vi "UHR-Fleezers Control (host) - Lorentz v5.vi"() -> ()   [LabVIEW 2014] (continued)
0.0016948540928536408, 0.004005193075967077, 0.000630961805097272, 0.0020857235483909497, 0.002248391411474813, 0.0025483315899778513, -0.00014289269800604444, 0.0013990991209830745, 0.002173222163707994, 0.0034697000160164738, 0.002010257683945241, 0.003481043985686529], [0.0018852656320276734, 0.0015715368380061585, 0.0019437671829601755, 0.002470975354509278, 0.0024487910797092428, 0.0007322022696453588, 0.0015475009764890752, 0.0017921866327059758, 0.003058459886432621, 0.0017764067983640703, 0.0025000139148490196, 0.0009623442611020518, 0.0018569165732802914, 0.003310838721775616, 0.00025071352576413444, 0.0036691347962582426, 0.002403046381925506, 0.004055721651469297, 0.002285952907609213, 0.0030062679778400502], [0.0024994380659973843, 0.0026197462346229062, 0.0017527989664171077, 0.0014375842896685127, 0.0033490362530976267, 0.0027052287063586847, 6.381847016474479e-05, 0.0011272327680753905, 0.003454975387457779, 0.004620127122907865, 0.0021178429445671146, 0.004539862151248757, 0.002029684806888378, 0.0013671243967539456, 0.003118446743148983, 0.0010709513970555225, 0.0019090166550763074, 0.002155844648949404, 0.004106378336132433, 0.0010766929367924097], [0.002854938319315421, 0.0038921928444872822, 0.0019246852509770592, 0.001956082424171971, 0.00249396489250124, 0.0024337273809226364, 0.0010765238019800384, 0.002941500719693421, 0.0030759660483101006, 0.0016202953746738819, 0.0017239866140603627, 0.002438327547432977, 0.002786814289877852, 0.002350374795189492, 0.0014284651785432274, 0.0024175263736445143, 0.0017989840672716986, 0.00010277744000073804, 0.0015758938162554312, 0.0015914808231177855], [0.0023379764512881855, 0.0019152406361689915, 0.0023721211744209382, 0.0028072318841611175, 0.00045998972816663626, 0.0019525984204332083, 0.001965702699358644, 0.0032523064679092764, 0.000928270862367026, 0.0025551238347956457, 0.0027235426100884804, 0.0006003323047511277, 0.0024452031525158107, 0.003200615692319165, 0.0031679408338207383, 0.001713752296656085, 0.0029069566496737467, 0.0017760622106257355, 0.0032846637736200987, 0.0014145046584398283], [0.0017413311095229888, 0.002850684453478228, 0.004119312336274303, 0.001376098161794153, 0.0028391954791758406, 0.0023504256794032296, 0.001939098372782241, 0.0009962144963960734, 0.0017508511614465492, 0.0010266285265010658, 0.00317450379791817, 0.002092576486750102, 0.003523745928434037, 0.003362704188893568, 0.0022223282833307503, 0.003285433624934814, 0.0021443498633667525, 0.0006378287745106628, 0.0009042965230192737, 0.004364189912157604], [0.0025684771943308964, 0.003595940600289024, 0.0015386127114892655, 0.002970017638684016, 0.000731008903710616, 0.0015627389249673368, 0.00268734680621615, 0.00033321301039761556, 0.002657761688265375, 0.0018452193301245214, 0.0019648865080461276, 0.00321862929090469, 0.002422721362346656, 0.0036160768033011536, 0.0023323715302130984, 0.0016526314538286777, 0.0033099223028642, 0.0014149263891099, 0.00254445644786201, 0.002714841511848489], [0.00302323496353701, 0.0016076200915618212, 0.001298400361326538, 0.0018074432822074325, 0.0026357010223677386, 0.002293142925429444, 0.001403310979000166, 0.002185113177831846, 0.002789454480226071, 0.0017208525559712065, 0.0017792513529249357, 0.0019822099798379907, 0.0028293142834817267, 0.002262865370925418, 0.001290800627866991, 0.0023298166748236485, 0.0013506602320411689, 0.002143358706259156, 0.0035532369528369174, 0.0017335871199569027], [0.0025192336907101567, 0.0023420394966944366, 0.0018803373952631193, 0.0019133833353522055, 0.0012596720449505453, 0.002147060132875675, 0.0006990538240453468, 0.0021223766921043765, 0.0033568805410328644, 0.0019950947049262504, 0.0021300391805659505, 0.001813624441258409, 0.0011352622065457982, 0.002742817450067307, 0.002825619560905981, 0.0028865080849197105, 0.003418778555540925, 0.0015302210369144652, 0.004455456383213908, 0.0013599469983302684], [-0.0004438837985084353, 0.0028183355707480946, 0.0028130708775573115, 0.0030206214884492544, 3.0807351233010224e-06, 0.00100356141409364, 0.003239142551743778, 0.0028015305417013713, 0.0016360555337629936, 0.0021630034342628546, 0.002737139846047398, 0.0036584890379432007, 0.002471730052534626, 0.0023361339599424456, 0.0029788411839639624, 0.0014442602794432905, 0.0023810759191331154, 0.0012413151489925564, 0.0019023668482100798, 0.002640107429201507], [0.001554782428247715, 0.002954419634687952, 0.0028951557424149637, 0.003310458814954959, 0.002365836700244099, 0.0030819547506098647, 0.0022846439376502706, 0.00043219002702368965, 0.003015949202071104, 0.002476214118282937, 0.0012666534517914985, 0.003753630460609294, 0.0019762301625312097, 0.0024128905675427107, 0.0024715495496260395, 0.0012053557199650255, 0.0030770984437811398, 0.001260030580666012, 0.002103542906975703, 0.003243844033696315], [0.002047169886274074, 0.003135570533130444, 0.003659218345652883, 0.003351918820368115, 0.002638669639842362, 0.0032054173808839705, 0.002728466251491257, 0.002422436287272547, 0.0027550251027393968, 0.0011484124718350213, 0.0024811181138690744, 0.000633754661919369, 0.004103389272200948, 0.002413442590560708, 0.0010161905814301843, 0.0006117013741451642, 0.00043229932014902874, 0.0026398449564406256, 0.002421923707756009, 0.0037337823125722382], [0.003223733537026557, 0.0018388836414569803, 0.0009593646694003638, 0.002150504738108695, 0.002240376826733987, 0.002819775892773071, 0.0023671589694118722, 0.000575767662750824, 0.002985254604568729, 0.0016894905303978737, 0.0022470149983889803, 0.0003279829367159081, 0.0036647064650229947, 0.0034208513812910607, 0.001372326074939035, 0.0012329776908317572, 0.0021677603380249777, 0.002634189260273172, 0.0028446181528041406, 0.00213113583206634], [0.0019954076065657263, 0.0037723924706211747, 0.001706529185397683, 0.002364821147683791, 0.002979725244773599, 0.0025437175845808863, 0.0021453554509108016, 0.004057319159369964, 0.003080980549531066, 0.002721994671347667, 0.0023390951175459806, 0.00256423096986864, 0.0028016019632848403, 0.004136674747509183, 0.0013482163844892154, 0.0025822615725757214, 0.0036704638004895884, 0.0027356369424274387, 0.0026386812531819896, 0.004017865052466032], [0.0024523481698112215, 0.001577397825690218, 0.003482073577677887, 0.0013120929321507693, 0.0023779996424196947, 0.0031885279055957677, 0.0030968142000769574, 0.0008079901646664205, 0.002057639245236158, 0.0014454916165466576, 0.0024913028609758626, 0.0037321652111583048, 0.0017568129726518262, 0.002433957686700396, 0.0013519635336044248, 0.0025583649394570035, 0.0028389004443714833, 0.0022371439658448768, 0.0027243471248494314, 0.0029988024916099377], [0.004482728416008117, 0.002106313095020212, 0.0016966090569018176, 0.002396355324914029, 0.0028921242144040655, 0.0015488778727110483, 0.003087584542752191, 0.0015783381053925663, 0.002107198839582597, 0.002028492535057995, 0.002133558230340132, 0.0033792319972435966, 0.0027693102835735124, 0.0018097134809963325, 0.0018729748671947632, 0.002639158100819596, 0.0020228765137224065, 0.0027609921089093853, 0.0018507896888375831, 0.0037945518126489184], [0.0021563482581923206, 0.0032287318120543937, 0.002708679733426596, 0.001050676702211846, 0.0025215820393785435, 0.0028877563801691696, 0.0019552140449292524, 0.0008869258799717261, 0.00135938852287414, 0.0018791457864769595, 0.0023044366557142164, 0.001505864205337834, 0.002869003954012599, 0.002875615556306393, 0.0002350922247605644, 0.001003648267132261, 0.002356427438894899, 0.0023482204070056395, 0.0030151148802336925, 0.0028427289795750045], [0.0038551731030675492, 0.0032190719566552277, 0.0024841888185482774, 0.0021509928606914825, 0.0019762178118407662, 0.0010938081355370294, 0.0013139616940169843, 0.0021720191912326476, 0.0022752909556785724, 0.001220901184309662, 0.0016582026045028472, 0.0024335127088734292, 0.0024787123106594982, 0.0020212943620039874, 0.0016344163085200308, 0.000406346466621824, 0.0029532673665144445, 0.0024979601850372486, 0.0026392577111319635, 0.004397563792842481], [0.0019392152337034533, 0.0025752001941428933, 0.002375394930020305, 0.0028141695664536765, 0.0030603007029344938, 0.0011131838617945628, 0.002016520759374347, 0.0007694648026350759, 0.0015220876353260865, 0.0007363225146947519, 0.000638103757805431, 0.0021367847621378373, 0.0006798563886399791, 0.0030144489262747447, 0.0012521090204634475, 0.0008366649244029356, 0.0025666821561406115, 0.001756081969563725, 0.0032417664621542308, 0.0027129101328840412], [0.004234965435631261, 0.0028807923900716586, 0.003994864856813696, 0.002228016783386847, 0.0020643224474904383, 0.0032080385730002244, 0.0024267095326168985, 0.0017045994219985895, 0.0004388872799201384, 0.0033081602061115307, 0.001876598014475262, 0.002967363816837642, 0.0014745477365160986, 0.0020882770356405143, 0.0013540441866247209, -0.0006440024187520807, 0.0028524616240076846, 0.0014866404270267755, 0.00212329751615424, 0.0033980422597344436], [0.002443103566818908, 0.0028643225076063544, 0.0026559502913978718, 0.0037632868164488202, 0.002284871036146773, 0.0015618259048538988, 0.0017562004198199274, 0.0013422612594893234, 0.0021296203269845397, 0.0025582835925385674, 0.0014546337054565813, 0.0012911088291717825, 0.0016512241182034806, 0.0022875704433646493, 0.003230826380294793, 0.0017297408349598563, 0.0026936683465980803, 0.0034380066316832677, 0.0020340691324621275, 0.0024417322062178165], [-9.989324566289746e-05, 0.002926244866839386, 0.0012902951621840647, 0.0026901742294294408, 0.0007707616757238599, 0.002362816916091356, 0.001011706400022051, 0.0017386970379252784, 0.0020217996444839735, 0.002564324057587132, 7.627346006863279e-05, 0.0002802241821891143, 0.0026582840805945995, 0.004267218692043419, 0.0008375444339060319, 0.001425992926040155, 0.0018555300552344036, 0.0019526652519745082, 0.0035856622760482276, 0.003574377792936731], [0.0022162866870525226, -9.80488992076956e-05, 0.0025575817989724257, 0.0017415298145425548, 0.0027732403933223874, 0.001805105566650088, 0.003135078437970281, 0.00030140619095551545, 0.002650648973281749, 0.0017502683903315023, 0.0010009292556551102, -0.0001580201494951381, 0.002096695649478786, 0.0023734494130614623, 0.001871656497385907, 0.0010147521269191551, 0.0028769559123858206, 0.001535512363638828, 0.0016771158914974686, 0.0036812015349025297], [0.0032911157382341976, 0.0015937673246648396, 0.0022786049298841506, 0.0016435202933210561, -0.000444139543920988, 0.0010322872285660274, 0.0015058197657779827, 0.0015226621305386731, 0.0013670575927993015, 0.001993129770992985, 0.0024129146141866654, -0.000271958439995209, 0.0032173265132192236, 0.001258442789528919, 0.0017013782876058627, 0.002937335820531526, 0.0020141218387929012, 0.00339081594854371, 0.0023237992039019865, 0.0019362936150417998], [0.0010726759952865783, 0.00383807561043779, 0.0038445499562823364, 0.0037327075782894294, 0.0030324176425392917, 0.000939469808843528, 0.0033586682713470056, 0.0007949762712558317, 0.0026842935481138233, 0.0027066995591428656, 0.001000126612503554, 0.0010644965226183879, 0.0012534863266311373, 0.000971090044070356, 0.0020274176610303746, 0.001313872990779878, 0.004415055089640197, 0.0022069739121942404, 0.000147794314328749, 0.003687654343198644], [0.0013238774283048135, 0.0016832656412011497, 0.002987102709259717, 0.0030815330868127306, 0.0029175865629059517, 0.001487872746945953, 0.0026091093679822507, 0.00135137082614052, 0.0011924192830799123, 0.002261800469194393, 0.000771417004330296, 0.0023250295522089758, 0.0016879132492112036, 0.0019726696926899378, 0.001788107104334166, 0.003862482787623552, 0.0024858537507722227, 0.00385855737054356, 0.0015301935270155484, 0.0031097752029073805], [0.0022271538965262065, 0.002149103591341216, 0.0008579581902112741, 0.0030474920826782247, 0.0032464784941930586, 0.002202404463612722, 0.0028610862175354876, 0.00119149906196459, 0.001159386660592406, 0.0010568905868378246, 0.0016045775757651311, 0.002078856957174876, 0.0031696706950223794, 0.0015400561930039819, 0.0018392034125027834, 0.0019016707318218183, 0.0025078250875444456, 0.0021647130900559666, 0.0006667868013903893, 0.002689612407972146], [0.003174915343868663, 0.0017082274160115402, 0.0004799123732484494, 0.002356906409014597, 0.002454123557174727, 0.0019283029529754366, 0.0005167238834184597, 0.0010390784903798918, 0.0022056908793985446, 0.0027450940851695103, 0.0015664249441001616, 0.0025970210907853447, 0.0031492312654002328, 0.0023489673010236925, 0.0016732664571149716, 0.0023468000185280606, 0.0006955608188309671, 0.0009160564453459453, 0.002208430013051778, 0.0010033313743313265], [0.002771809170291859, 0.0013473649729025135, 0.0020308167485843616, 0.0033787301181636546, 0.00265669183861397, 0.002015256758420677, 0.0021247098216520435, 0.001977968519838654, 0.0034117189837875477, 0.0017658010805061703, 0.0025104575542475244, 0.002180588571631346, 0.0027725271015961524, 0.0036683916030291934, 0.00346879977795831, 0.0016237785338239006, 0.0013883707480767996, 0.0030502992866057047, 0.0031019819698129046, 0.0016354795807633777]]
  in  "Channel":i32=4
  in  "Abort MCL Scan":bool
  out "MCL Scan I":u64
  out "MCL Scanning":bool
  in  "Start MCL Scan":bool
  out "wait to reset values":bool
  in  "Tab Control 4":enum32{"Scan Settings", "MCL FPGA Loop Timing"}(tab)
  out "Total Time (s)":dbl=4.8
  in  "Scan lines (y)":u64=20
  in  "Fast Scan Dir":bool=TRUE
  in  "2D or 1D Scan":bool=TRUE
  out "Initial X":dbl=1.3285729544969032
  out "Initial Y":dbl=4.00431745353557
  out "Time/f+b scan (s) (MCL)":dbl=0.24 caption="Time/scan (s)"
  in  "Number of scans (MCL)":u64=1 caption="Scans"
  in  "Scan steps (MCL)":u64=40 caption="Scan steps (x)"
  in  "N APD Samp/step":dbl=3.0
  in  "Scan Range (V)\n(of steps)":dbl=7.0
  in  "Restart DMA? (MCL)":bool=TRUE caption="Restart DMA?"
  in  "Continuous MCL Scanning":bool caption="Cont. Scanning"
  in  "Center Scan":bool=TRUE
  in  "Save Data (MCL)":bool=TRUE caption="Save Data"
  out "Actual Incr. int (MCL)":i16=588 caption="Incr. int"
  out "Desired incr (int)":dbl=588.125641025641
  out "Desired Scan Incr (V)":dbl=0.1794871794871795
  out "N sets should be saved (MCL)":dbl=16.0 caption="N sets should be saved"
  out "Data points/scans (MCL)":dbl=4800.0 caption="Data points/scans"
  out "Data points/scan (f+b)":dbl=240.0 caption="points/scan (f+b)"
  out "Cycles/step (MCL)":u64=300 caption="Cycles/step" format="%.0p"
  out "Actual MCL Inc (V)":dbl=0.1794488357188635
  in  "Phase adjust (MCL)":i16 caption="Phase adjust"
  out "Relative Phase (MCL)":i16 caption="Relative Phase"
  in  "Initial Phase Adj. (MCL)":i16 caption="Initial Phase Adj."
  in  "Update Count (MCL)":u32=400
  in  "+ phase (MCL)":bool
  in  "- phase (MCL)":bool
  out "MCL Late Counter":u8
  in  "APD AO Scale Factor":i16=1 min=1
  in  "Fluorescent excitation laser controls":T21(tab)
  in  "Interlace OFF count":u16=450 min=1 step=1
  in  "Interlace ON count":u16=150 min=1 step=1
  in  "Duty Frequency (ON 1/N cycles)":u16=1
  in  "Invert laser interlacing":bool
  out "Fluorescence laser intensities plot":cluster{dbl, dbl, dbl}(graph)
  in  "Green FB On/Off":bool
  in  "Red FB On/Off":bool
  in  "Blue FB On/Off":bool
  in  "Red Intensity % (FB OFF)":dbl=20.0 min=0.0 max=100.0 step=1.0
  in  "Blue Intensity % (FB OFF)":dbl=87.0 min=0.0 max=100.0 step=1.0
  out "Green laser intensity (V)":dbl
  in  "Initial Phase Adjustment (Green FB)":i16=-30
  in  "Phase adj. (Green FB)":i16=10
  out "Green AI Count":u16=600
  in  "- phase (Green FB)":bool
  in  "+ phase (Green FB)":bool
  out "Relative phase (Green FB)":i16
  out "GI Late Counter 2":u8
  in  "Phase adj. (GI) 2":i16=1
  out "GI relative phase 2":i16
  in  "+ phase (GI) 2":bool
  in  "Initial Phase Adjustment (GI) 2":i16=-274
  in  "- phase (GI) 2":bool
  in  "Green FB Gains":T14={"proportional gain (Kc)"=10, "integral gain (Kc*Ts/Ti)"=5, "derivative gain (Kc*Td/Ts)"=0}
  in  "Green int current ON count adj":u32=150
  in  "- phase (GI)":bool
  in  "Initial Phase Adjustment (GI)":i16=-28
  in  "+ phase (GI)":bool
  out "GI relative phase":i16
  in  "Phase adj. (GI)":i16=1
  out "GI Late Counter":u8
  out "Green AI Late Counter":u8
  out "MCL Scan":cluster{"Begin (V)":dbl, dbl, dbl[]}(graph)
  out "MCL Scan 2":cluster{"Begin (V)":dbl, dbl, dbl[]}(graph)
  out "Red laser intensity (V)":dbl
  out "Red AI Count":u16=600
  in  "Initial Phase Adjustment (RI)":i16=25
  out "RI Late Counter":u8
  in  "Red FB Gains":T14={"proportional gain (Kc)"=10, "integral gain (Kc*Ts/Ti)"=5, "derivative gain (Kc*Td/Ts)"=0}
  in  "Phase adj. (RI)":i16=20
  out "RI relative phase":i16
  in  "+ phase (RI)":bool
  in  "- phase (RI)":bool
  in  "Blue Laser Modulation Mode":string(combo)
  out "Digital Modulation":bool
  out "Analog Modulation":bool
  out "Laser On":bool
  in  "Get Blue Laser State":bool
  out "Blue laser intensity (V)":dbl
  out "Relative phase (BI AO)":i16
  out "Relative phase (BI DO)":i16
  out "Late Counter (BI DO)":u8
  out "Late Counter (BI AO)":u8
  in  "Initial Phase Adjustment (BI DO)":i16=65
  in  "Initial Phase Adjustment (BI AO)":i16
  in  "Phase adj. (BI AO)":i16=20
  in  "+ phase (BI AO)":bool
  in  "- phase (BI AO)":bool
  in  "Blue int AO ON count adjust":u16=150
  in  "Blue FB Gains":T14={"proportional gain (Kc)"=10, "integral gain (Kc*Ts/Ti)"=5, "derivative gain (Kc*Td/Ts)"=0}
  in  "- phase (BI DO)":bool
  in  "+ phase (BI DO)":bool
  in  "Phase adj. (BI DO)":i16=20
  out "Blue AI Count":u16=600
  in  "Delay (ms)":i32=500
  in  "Send string\nto Blue Laser":bool
  in  "command string":string
  out "command string sent":string="sames 0"
  out "read blue buffer":string
  out "Blue Error Out":errorcluster={"status"=TRUE, "code"=-1073807346, "source"="VISA Write in serial write macro.vi->UHR-Fleezers Control (host) - Lorentz v5.vi"}
  in  "VISA resource name":refnum<visa-resource-name>="Blue-Laser-COM7"
  in  "Blue Laser Modulation\nPower (mW)":string="80"
  in  "Blue Laser Power (mW)\n(Constant Power Mode)":string="70"
  in  "Flip X Sign":bool=TRUE
  in  "Trap Position FIFO Depth":u32=300000 format="%.0p"
  in  "# Samples/trap":u32=20000
  out "Trap AI Elements/DMA read":u32=320000 format="%.0p"
  out "Ave. Rate (Hz)":dbl=200000.0 format="%#_6p"
  out "FIFO El. Rem.":u32=3 format="%.0p"
  in  "Phase adj. (AI1)":i16=10
  out "Relative phase (AI1)":i16=-170
  in  "+ phase (AI1)":bool
  in  "- phase (AI1)":bool
  out "Late Counter (AI1)":u8
  in  "Initial Phase Adjustment (AI1)":i16=170
  out "AI rate (Hz)":dbl=200000.0 format="%#_6p"
  in  "AI Count (ticks)":u16=200
  out "# Samples/channel":u32=40000 format="%.0p"
  in  "Trap AI FIFO Depth":u32=900000
  in  "Detector Type":string(combo)="IR-QPD + PSD + FB-QPD X position"
  in  "N Acq Sets (Traps + Fl.)":i16=2
  in  "Sets to FIFO (Traps)":T22={"Set 1"=TRUE, "Set 2"=TRUE, "Set 3"=FALSE}
  in  "FPGA Ave.":dbl=1.0 min=1.0 step=1.0
  out "Ave. Period (s)":dbl=5e-06 format="%#_6p"
  out "DMA Update Period (s)":dbl=0.2
  out "FPGA Averaging":bool
  out "Trap Sets":u32=2
  out "Counts/DMA":dbl=8000000.0 format="%#_6p"
  out "Trap Pos FIFO El Remaining":u32=3425 format="%.0p"
  out "Trap Pos Elements/DMA read":u32=200000 format="%.0p"
  out "Trap AI FIFO Timeout":u16
  out "Trap Pos FIFO Timeout":u16
  out "error out":errorcluster
  out "error out 2":errorcluster
  in  "Piezo trap 0 position relative to 75 MHz":cluster{"X (V)":dbl, "Y (V)":dbl}={"X (V)"=3.0, "Y (V)"=0.0}
  in  "Piezo Trap Y cal (nm/V)":dbl=200.0
  in  "Piezo Trap X cal (nm/V)":dbl=200.0
  in  "Bottom  1 Harvard Syringe Pump Serial Port":refnum<visa-resource-name>="Bottom-Pump1-COM5"
  in  "Center Harvard Syringe Pump Serial Port":refnum<visa-resource-name>="Central-Pump2-COM6"
  in  "Lost Tether Alarm Threshold (pN)":dbl=0.5
  in  "AOM X Cal (nm/MHz)":dbl=200.0
  in  "MCL X Cal (nm/V)":dbl=739.5
  out "X RF Amplitude Limits (%)":T23={"Minimum"=0.0, "Maximum"=50.0, "Increment"=1.0}
  out "X RF Frequency Limits (MHz)":T23={"Minimum"=60.0, "Maximum"=90.0, "Increment"=1.0}
  out "Y RF Frequency Limits (MHz)":T23={"Minimum"=0.0, "Maximum"=40.0, "Increment"=0.1}
  out "Y RF Amplitude Limits (%)":T23={"Minimum"=0.0, "Maximum"=45.0, "Increment"=1.0}
  in  "Manip. X?":bool=TRUE
  in  "Manip. Y?":bool
  in  "Force Manip Abort":bool
  out "Read cal error":errorcluster={"status"=TRUE, "code"=7, "source"="Open/Create/Replace File in UHR-Fleezers Control (host) - 15.2.1UCBMengV9.vi<APPEND>\nP:\\Data\\160111\\current.cal"}
  in  "DAQ Delay (ms)":u32=1000
  in  "Start Scan":bool
  in  "Scan axis":bool=TRUE
  in  "Osc. amp. (V)":dbl=5.0
  in  "Osc. center (V)":dbl=5.0
  in  "Osc. freq. (Hz) 2":dbl=1.0
  in  "MCL Mode":u16(ring) items=["Manual Positioning", "Sinusoidal Wave", "Linear Scan"]
  in  "Begin (V)":dbl
  in  "End (V)":dbl=10.0
  in  "N Points":dbl=20.0
  in  "Delay to Interlace (s)":dbl
  in  "Delayed Interlace Start":bool
  in  "Read Lateness and Rel Phase":bool=TRUE
  out "Vec Mean of T1 T2":dbl[](array[numeric])
  in  "Cal read wait (s)":u32=5
  out "Time tether formed":timestamp=timestamp(3534521622.0325327 s since 1904-01-01)
  in  "Sample Chamber Stage Serial Port":refnum<visa-resource-name>="Sample-Stage-COM1"
  in  "Chemyx Syringe Pump Serial Port":refnum<visa-resource-name>="ASRL3::INSTR"
  in  "Limit Min (MHz)":dbl=10.0 caption="Min (MHz)"
  in  "Limit Max (MHz)":dbl=16.0 caption="Max (MHz)"
  in  "Limits Enable":bool=TRUE caption="Enable"
  out "AI labels":string[](array[string])=["T1 Y", "T1 X", "T1 Sum", "T2 Y", "T2 X", "T2 Sum", "T1 FB X", "T1 FB Sum", "T2 FB X", "T2 FB Sum", "T3 Y/ PSD Y", "T3 X / PSD X", "T3 Sum / PSD sum"]
  in  "Save Trap Pos. Data":bool=TRUE
  in  "Lower Ch. Cap.":bool
  in  "Top 3 Harvard Syringe Pump Serial Port":refnum<visa-resource-name>="Top-Pump3-COM4"
  out "Database link":path=path "C:/Home/Bustamante Lab/Comstock-LabView-Link.udl"
  out "connection reference":T24
  out "FPGA error out":errorcluster
  out "Trigger Signal":dbl[](graph)=[1.953852737276498, 1.8613052147403675]
  in  "Fish mask thresh":dbl=0.5
  in  "Normal (on) or masked test (off)":bool=TRUE
  in  "Stop F (pN) (mask)":dbl=1.0
  in  "Osc. freq. (Hz)":dbl=0.25
  in  "Trap shift\nmethod":bool=TRUE
  in  "Pause rotation":bool
  out "Waveform Chart":dbl(graph)
  in  "Trap 2 phase shift (deg)":dbl caption="Fixed phase shift (deg)"
  in  "Radius (MHz)":dbl=2.0 min=0.0 max=10.0 step=0.1
  out "Trap trajectories":cluster{dbl[], dbl[]}[](graph)
  in  "Move in a Circle":bool
  in  "Center Y Frequency (MHz)":dbl=31.0
  in  "Stop Moving":bool
  in  "2D Motion Frequency (Hz)":dbl=0.25
  in  "2D Motion Trap Separation (MHz)":dbl=0.75 caption="Fixed distance (MHz)" min=0.0 max=10.0 step=0.1
  in  "Time step (ms)":i64=10
  in  "N steps then stop":i32
  in  "Back to start on finish?":bool=TRUE
  in  "Counterclockwise/Clockwise":bool
  out "Trap 1 sum mean":dbl=-0.09989539366334516 format="%0.2f"
  out "Trap 2 sum mean":dbl=-0.06614011795561298 format="%0.2f"
  in  "index 1":i32=3
  in  "index 2":i32
  in  "test":bool
  in  "Reset graph":bool
  in  "N steps to plot":i32=1000
  out "Waveform Graph 2":waveform(dbl)(graph)
  in  "Offset 2":dbl
  in  "mult x":dbl
  in  "Offset":dbl
  out "N data samples":dbl
  out "Initial buffer time (s)":dbl
  in  "N initial buffer elements":u16=5000
  in  "Sound ON":bool
  in  "Carrier Frequency (Hz)":dbl=300.0
  in  "number of samples/ch":i32=100000
  in  "sample mode":T25=1 items=["Finite Samples", "Continuous Samples"]
  in  "device ID":u32
  in  "sound format":T26={"sample rate (S/s)"=22050.0, "number of channels"=2, "bits per sample"=16}
  in  "Volume":dbl=1.0 format="%0.2p"
  in  "interpolation mode":u16(ring)=1 items=["coerce", "linear", "spline", "FIR filter"]
  in  "tone or data":bool
  in  "Data channel to sound":i32
  in  "Base N trap periods":u32=50
  in  "Period scale factor":dbl=4.0
  in  "Trap osc amp (MHz)":dbl=1.0
  in  "Osc trap cont.":bool
  in  "Osc traps":bool
  out "Trap OSC Period (s)":dbl=0.002
  out "Writing waveform to fpga memory":bool
  in  "Save trap pos with cal":bool=TRUE
  in  "T1 Osc Enable":bool=TRUE
  in  "T2 Osc Enable":bool=TRUE
  out "DMA remainder":u64
  out "(total save/100) /osc period remainder":u32
  out "Total save/100 remainder":u32
  out "N osc/ (total save/100)":u64=25
  out "N osc / DMA":u64=100
  out "N trap osc periods per save":u64
  out "N trap osc periods per save remainder":u64
  in  "Command":string
  out "Reply":string
  in  "Send Command":bool
  out "Preamp Error Out":errorcluster
  in  "Gain Mode":string(combo)="0"
  in  "Invert Signal":bool
  in  "Sensitivity":string(combo)="0"
  in  "Offset Current Sign":bool=TRUE
  in  "Offset Current Value":string(combo)
  in  "Offset Current":bool
  in  "Bias Voltage":bool
  in  "Bias Voltage (mV)":i32
  in  "Filter Type":string(combo)="4"
  in  "Lowpass 3dB Point":string(combo)="6"
  in  "Highpass 3dB Point":string(combo)
  in  "Filter Reset":bool
  out "Command Sent":string
  out "Gain":string(combo)="0"
  # "X"
  # "Y"
  # "Data Saving"
  # "External fluorescence triggering tests:"
  # "After"
  # "During"
  # "Trap On?"
  # "BD Flow ON?"
  # "Samp Flow ON?"
  # "Trap Trig. Fl.?"
  # "Zero It"
  # "Floor it\n(e.g., hp unwinding)"
  # "1"
  # "2"
  # "Fl. Down"
  # "Fl. Up"
  # "T1 Y"
  # "T1 X"
  # "T1 Sum"
  # "T2 Y"
  # "T2 X"
  # "T2 Sum"
  # "FB1 X"
  # "FB1 Sum"
  # "FB2 X"
  # "FB2 Sum"
  # "T3 Y"
  # "T3 X"
  # "T3 Sum"
  # "Trap Display:"
  # "APD Display:"
  # "DAQ"
  # "Trap Manipulation"
  # "Bead Calibration"
  # "MCL trap"
  # "Fine Motor Control"
  # "Bottom Pump (#1)"
  # "Central Sample Channels"
  # "Top Pump (#3)"
  # "Rate param is ul/h\nVolume param is ul"
  # "Chemyx Pump 2"
  # "Units: \n1 = ml/m\n2 = ml/h\n3 = ul/m\n4 = ul/h"
  # "Choose method of updating trap RF values: false is usual, true is use external loop method\n(in order to increase possible delay between X and Y signals -- to synchronize X and Y switching)"
  # "Delay to switch frequency and amplitude of boards.\nUsed to align phases of boards (finely)."
  # "X"
  # "Y"
  # "Oscillate Set 1 freq. (debugging)"
  # "BD 1"
  # "BD 2"
  # "Amp switch 1st is disabled in the fpga!\nSeems its also frequency that needs to go first (for all boards tested so far)."
  # "AOD Raster Scan"
  # "Approx. trap separations"
  # "X"
  # "Y"
  # "FPGA\nreading"
  # "DMA\ntransfer"
  # "APD Integration Loop"
  # "APD Gates"
  # "APD 2 (Cy5)"
  # "APD 3 (Cy2)"
  # "APD 1 (Cy3)"
  # "X"
  # "2D"
  # "Y"
  # "1D"
  # "Digital Out Control"
  # "Analog Out Control (Feedback Loop)"
  # "Laser Intensity Analog Input"
  # "Operational note:\n\nUse the digital out control to adjust red laser\ntiming (fine tuning).\n\nAt the moment, the red laser analog out\ncontrol timing is identical and set by green \nlaser AO timing (in the same loop).  Otherwise\nyou can not get synchronous timing with the\ncurrent AO expansion board.\n\nSimilarly, the AI measurement is also \nsimultaneous for all three lasers (for the same\nreason).\n\nThese controls are kept for possible future\nuse."
  # "Analog Out Control (Feedback Loop)"
  # "Digital Out Control"
  # "Laser Intensity Analog Input"
  # "Operational note:\n\nThe AI measurement is simultaneous for all three lasers\n(see red laser note).\n\nThese controls are kept for possible future use."
  # "Analog Out Control (Feedback Loop)"
  # "Laser Intensity Analog Input"
  # "Digital Out Control"
  # "Total AI Rates (NOT rates/trap)"
  # "(Samples/trap x Trap Sets)"
  # "(Samples/channel x\n8 if averaging (8 channels)\n4 if no averaging)"
  # "Trap 1"
  # "Trap 2"
  # "Flour./Trap 3"
  # "External Video Window"
  # "3: IR LED\n2: Blue LED"
  # "MCL Position Debugging"
  # "Temporary Control Storage\n(these used to be somewhere else, still want to keep them)"
  # "Database config"
  # "Y"
  # "X"
  # "Trap Position Difference Limits"
  # "Start trapping above center (> center MHz)\n\nNegative trap separation means trap 2 follows\n(starts to the right)"
  # "Initialization"
  # "Radius initially determined by center\nand current location (then can be changed)"
  # "Active (oscillating) trap calibration:"
  # "All these remainders\nshould be 0."
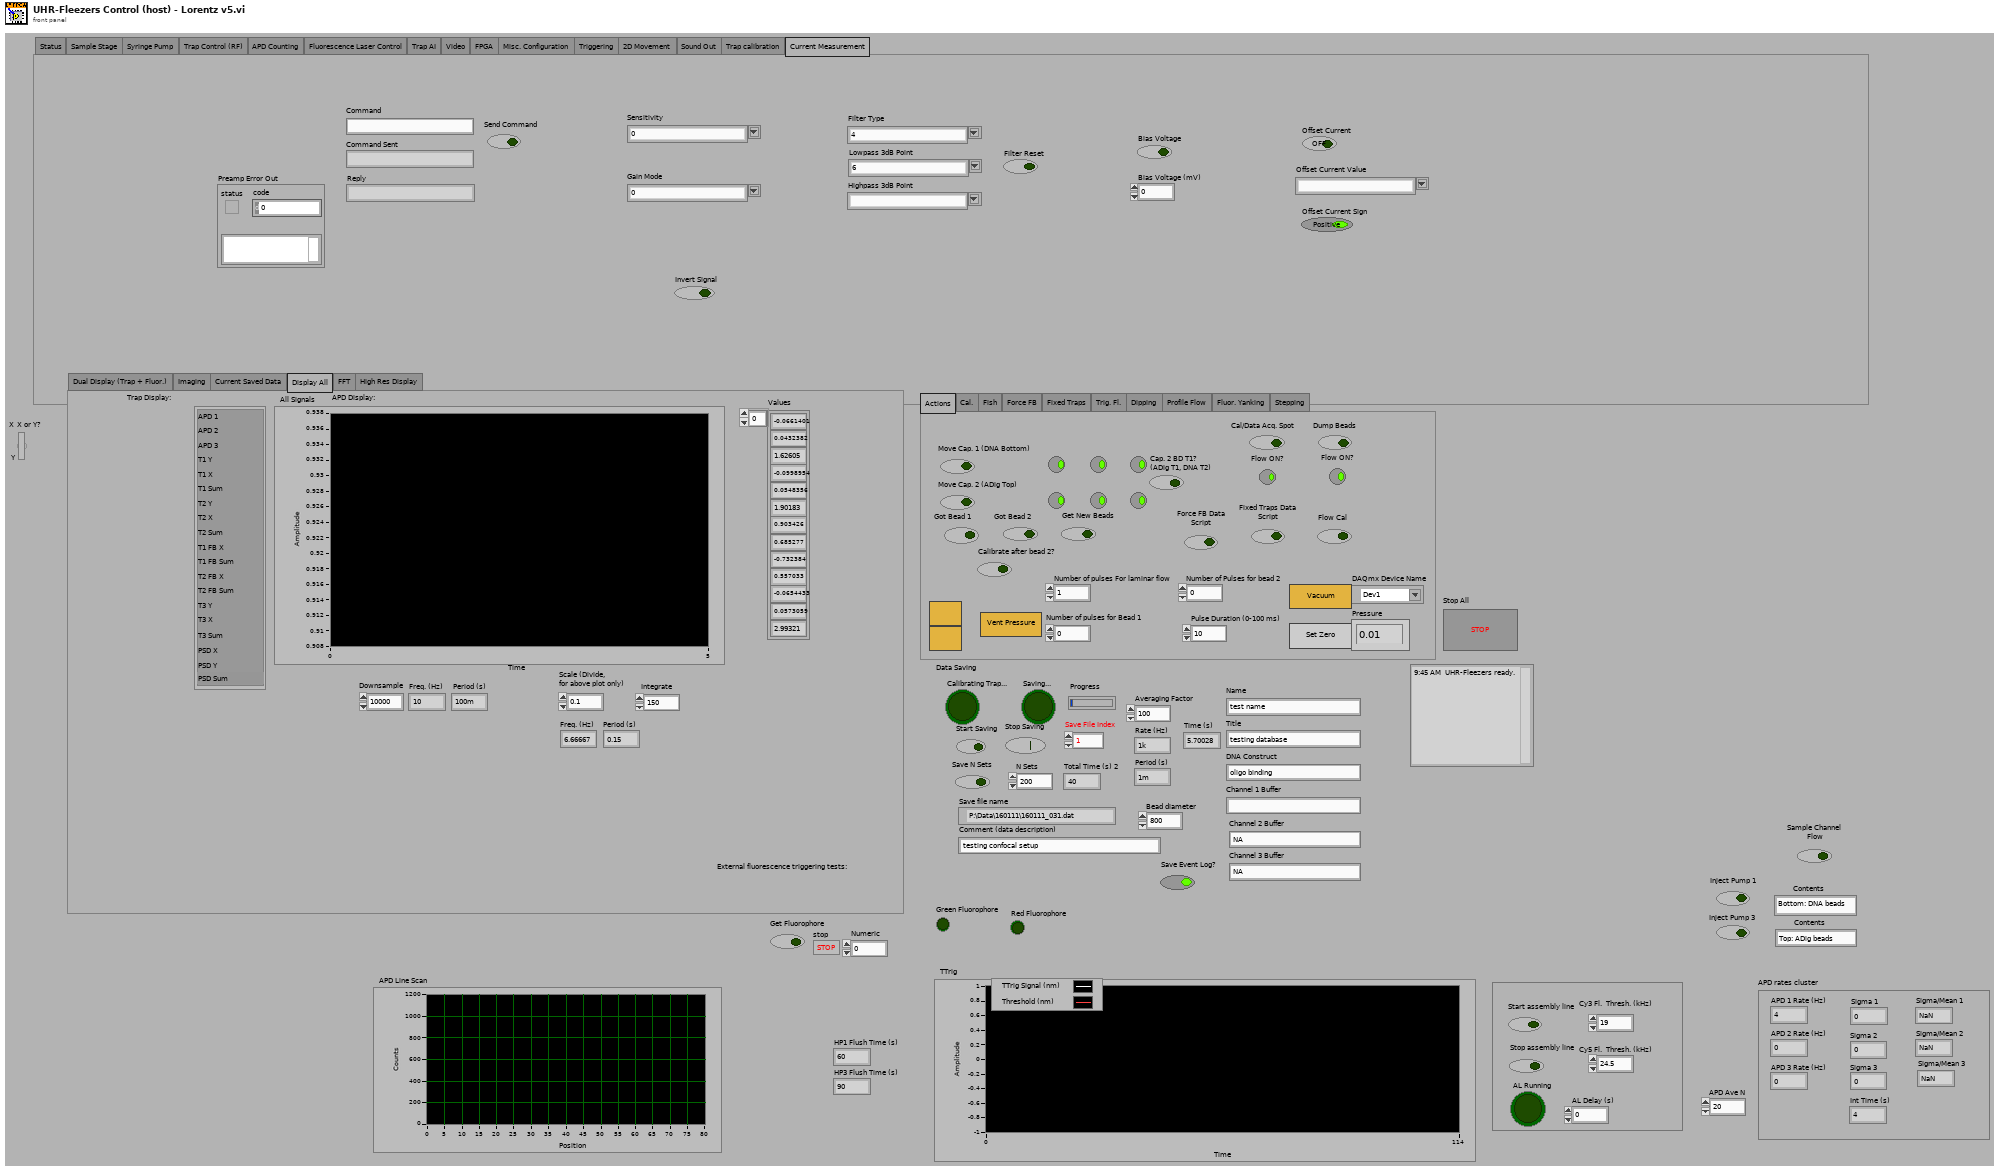
[diagram p1: front panel]
types:
  T1 = cluster{"APD 1 Rate (Hz)":dbl, "APD 2 Rate (Hz)":dbl, "APD 3 Rate (Hz)":dbl, "Sigma/Mean 1":dbl, "Int Time (s)":dbl, "Sigma 1":dbl, "Sigma 2":dbl, "Sigma 3":dbl, "Sigma/Mean 2":dbl, "Sigma/Mean 3":dbl}
  T2 = enum32{"Actions", "Cal.", "Fish", "Force FB", "Fixed Traps", "Trig. Fl.", "Dipping", "Profile Flow", "Fluor. Yanking", "Stepping"}
  T3 = enum32{"Dual Display (Trap + Fluor.)", "Imaging", "Current Saved Data", "Display All", "FFT", "High Res Display"}
  T4 = cluster{"T1 X":dbl, "T2 X":dbl, "T3 X":dbl, "T3 Y":dbl}
  T5 = cluster{"T1 X":bool, "T2 X":bool, "T3 X":bool, "T3 Y":bool}
  T6 = typedef "IMAQ Image.ctl" = refnum<image>
  T7 = enum32{"Status", "Sample Stage", "Syringe Pump", "Trap Control (RF)", "APD Counting", "Fluorescence Laser Control", "Trap AI", "Video", "FPGA", "Misc. Configuration", "Triggering", "2D Movement", "Sound Out", "Trap calibration", "Current Measurement"}
  T8 = cluster{"T2 alpha_x (nm/V)":dbl, "T2 offset_x (mV)":dbl, "T2 kappa_x (pN/nm)":dbl}
  T9 = cluster{"T1 alpha_x (nm/V)":dbl, "T1 offset_x (mV)":dbl, "T1 kappa_x (pN/nm)":dbl}
  T10 = cluster{"Pump 1":cluster{"Diameter (mm)":dbl, "Units":dbl, "Volume":dbl, "Rate":dbl}, "Pump 2":cluster{"Diameter (mm)":dbl, "Units":dbl, "Volume":dbl, "Rate":dbl}, "Pump 3":cluster{"Diameter (mm)":dbl, "Units":dbl, "Volume":dbl, "Rate":dbl}}
  T11 = enum32{"IR Laser Interlacing (Direct RF Board Control Method)", "AOD Raster Scan", "Feedback on Trap Intensity", "Feedback on Trap Position"}
  T12 = typedef "LVPoint32TypeDef.ctl" = cluster{"Horizontal":i32, "Vertical":i32}
  T13 = cluster{"Scan Range AOD (nm) 2":dbl, "Step Size AOD (nm) 2":dbl, "Scan Speed AOD (nm/s) 2":dbl, "Number of scans (AOD) 2":u16, "Label":string}[]
  T14 = cluster{"proportional gain (Kc)":i16, "integral gain (Kc*Ts/Ti)":i16, "derivative gain (Kc*Td/Ts)":i16}
  T15 = cluster{"Trap 1":fxp<+/-,16,1>, "Trap 2":fxp<+/-,16,1>}
  T16 = enum32{"Main Setting", "Details", "Dynamic FB settings", "Semi Passive Mode"}
  T17 = cluster{"proportional gain (Kc)":fxp<+/-,16,8>, "integral gain (Kc*Ts/Ti)":fxp<+/-,16,8>, "derivative gain (Kc*Td/Ts)":fxp<+/-,16,8>}
  T18 = cluster{"output high":fxp<+/-,16,1>, "output low":fxp<+/-,16,1>}
  T19 = cluster{"Set 1":fxp<+/-,16,1>, "Set 2":fxp<+/-,16,1>}
  T20 = cluster{"Trap 1X offset":dbl[], "Trap 2X offset":dbl[]}
  T21 = enum32{"Main Controls", "Green laser (532 nm)", "Red laser (633 nm)", "Blue laser (473 nm)"}
  T22 = cluster{"Set 1":bool, "Set 2":bool, "Set 3":bool}
  T23 = typedef "LVMinMaxIncTypeDef.ctl" = cluster{"Minimum":dbl, "Maximum":dbl, "Increment":dbl}
  T24 = typedef "NI_Database_API.lvlib/Conn ObjectReference.ctl" = refnum<k1>
  T25 = typedef "Sampling Mode.ctl" = i32
  T26 = typedef "Sound Data Format.ctl" = cluster{"sample rate (S/s)":dbl, "number of channels":i32, "bits per sample":i32}
  T27 = typedef "nirio_resource_hc.ctl" = tag
  T28 = typedef "Image Type" = u32
  T29 = typedef "Pressure Control.lvclass/Pressure Control Config.ctl" = cluster{"daqmx_channel":string, "terminal_configuration":string}
  T30 = cluster{string, "TTL line # Pressure Up":u8, bool, bool}
  T31 = cluster{string, "TTL line # Pressure Down":u8, bool, bool}
  T32 = cluster{string, "TTL line # Pressure Vacuum":u8, bool, bool}
  T33 = cluster{string, "TTL line # Pressure Vacuum":u8, bool, bool}[]
  T34 = cluster{"New Image":T6, "New Image":T6, "New Image":T6, "New Image":T6, "New Image":T6}
  T35 = typedef "openfpgaref.8.6.ctl" = refnum<k20>
  T36 = typedef "XDNodeRunTimeDep.lvlib/timing_clust.ctl" = cluster{"Expected End [f-1]":u64, "Actual End [f-1]":u64, "Finished Late? [f-1]":bool, "Expected End [i-1]":u64, "Actual End [i-1]":u64, "Finished Late? [i-1]":bool, "Expected Start [i]":u64, "Actual Start [i]":u64, "Expected Start [f]":u64, "Actual Start [f]":u64, "Source Name":string, "Structure Name":string, "Period":i64, "Deadline":i64, "Offset":i64, "Start":i64, "Priority":i32, "Timeout":i32, "Mode":T37, "Wakeup Reason":T38, "Error":errorcluster, "Source Type":string, "Secondary Source Type":string, "Global End Time":u64, "Global Start Time":u64, "Frame Duration":u64, "Iteration Duration":u64, "Assigned CPU":i32, "I/O Scan Engine Mode":u32}
  T37 = typedef "XDNodeRunTimeDep.lvlib/nitl_modes.ctl" = enum32{"No Change", "Process missed periods, maintain original phase", "Discard missed periods, maintain original phase", "Process missed periods, ignore original phase", "Discard missed periods, ignore original phase"}
  T38 = typedef "XDNodeRunTimeDep.lvlib/wakeup.ctl" = enum32{"Normal", "Aborted", "Asynchronous wakeup", "Timing source error", "Timed loop error", "Timeout"}
  T39 = enum32{"Status", "Sample Stage", "Syringe Pump", "Trap Control (RF)", "APD Counting", "Fluorescence Laser Control", "Trap AI", "Video", "FPGA"}
  T40 = enum32{"Status", "Sample Stage", "Syringe Pump", "Trap Control (RF)", "APD Counting", "Fluorescence Laser Control", "Trap AI", "Video", "FPGA", "Misc. Configuration"}
  T41 = enum16{"CONNECT", "INITIALIZE VALVES", "DISCONNECT", "MOVE VALVE"}
  T42 = enum16{"empty", "write", "read oldest (queue)", "read newest (stack)", "read all"}
  T43 = enum16{"open", "replace", "create", "open or create", "replace or create", "replace or create with confirmation"}
  T44 = enum16{"big-endian, network order", "native, host order", "little-endian"}
  T45 = cluster{"Scan Range AOD (nm) 2":dbl, "Step Size AOD (nm) 2":dbl, "Scan Speed AOD (nm/s) 2":dbl, "Number of scans (AOD) 2":u16, "Label":string}
  T46 = cluster{"[0]":dbl, "[1]":dbl, "[2]":dbl, "[3]":dbl, "[4]":dbl, "[5]":dbl}
  T47 = cluster{"Diameter (mm)":dbl, "Units":dbl, "Volume":dbl, "Rate":dbl}
  T48 = cluster{"Left":i32, "Top":i32, "Width":u32, "Height":u32}
  T49 = cluster{cluster{"Left":i32, "Top":i32, "Width":u32, "Height":u32}}[]
  T50 = typedef "Sound Output Task ID.ctl" = u32
  T51 = enum32{"Normal Display", "Dual Display (APD)", "FFT", "High Res Display"}
  T52 = cluster{"Origin Pixel":cluster{"X":sgl, "Y":sgl}, "Angle Relative to Horizontal (deg)":sgl, "Axis Reference":u32}
  T53 = typedef "Simple Grid Descriptor" = cluster{"X Step":sgl, "Y Step":sgl, "Unit":T54}
  T54 = typedef "Image Unit" = enum32{"Undefined", "Angström", "Micrometer", "Millimeter", "Centimeter", "Meter", "Kilometer", "Microinch", "Inch", "Feet", "Nautical miles", "Standard miles", "Steps"}
  T55 = cluster{"averaging mode":u16, "weighting mode":u16, "number of averages":u32}
  T56 = cluster{"dB On (F)":bool, "unwrap phase (F)":bool, "convert to degree (F)":bool}
  T57 = cluster{"Scan Range (nm)":dbl, "MCL Step Position Ratio":dbl, "MCL/AOM Scale Tweak":dbl, "MCL X Cal (nm/V)":dbl, "MCL Step Increment (V_int)":dbl, "Total Counts (ticks)":u16, "Scan steps (AOD)":u64, "Cycles/step (AOD)":u64}
  T58 = cluster{"Actual MCL Inc (V)":dbl, "Scan steps (MCL)":u64, "Scan lines (y)":u64, "AO1":dbl, "AO2":dbl}
  T59 = cluster{"APD 1":u32[], "APD 2":u32[], "APD 3":u32[]}
  T60 = cluster{"RMS[0]":dbl, "RMS[1]":dbl, "RMS[2]":dbl, "RMS[3]":dbl}
  T61 = cluster{"Mean [0]":dbl, "Mean [1]":dbl, "Mean [2]":dbl, "Mean [3]":dbl}
  T62 = cluster{"f0":dbl, "df":dbl, "magnitude":dbl[]}[][]
  T63 = cluster{"Comment (data description)":string, "Channel 1 Buffer":string, "Channel 2 Buffer":string, "Channel 3 Buffer":string, "Title":string, "DNA Construct":string, "Bead diameter":dbl, "Name":string}
diagram:
  w4 = 90.0
  w32 = T28 2 items=["Grayscale (U8)", "Grayscale (I16)", "Grayscale (SGL)", "Complex (CSG)", "RGB (U32)", "HSL (U32)", "RGB (U64)", "Grayscale (U16)"] ("Image Type")
  # "X limits"
  # "Amp Lmits"
  # "Freq Limits"
  # "Changed by Ronen - All events relating to activation of the pumps have been disabled: 56, 55, 54, 53, 52, 51, 50, 49, 48, 47, 46, 45, 44, 43, 41, 40"
  # "Harvard Pump control disabled by Hendrik"
  # "Settings to help prevent AOM/D damage"
  # "Initialize the FPGA DAQ card itself"
  # "Reset the DAQ card."
  # "Specify the DAQ card and the FPGA code to run"
  # "Bottom 1 Harvard"
  # "Top 3 Harvard"
  # "Center Harvard"
  n1 = disable-structure shown="Enabled" {
    frame Enabled {
      w102 = FALSE
      # "This Control added by\nRonen to enable direct\nControl of pressure pulse\nlength to enable fine flow\ncontrol"
      # "Start out with all lines set to zero"
      n2 = Format Into String(format string="%s/port0/line5:1, %s/port1/line0:3", "DAQmx Device Name", "DAQmx Device Name") -> (resulting string=w94:string)  [unwired: 2 in, 1 out]
      n3 = Format Into String(format string="%s/ai0", "DAQmx Device Name") -> (resulting string=w92:string)  [unwired: 2 in, 1 out]
      n4 = In Range and Coerce(upper limit=100.0, x="Pulse Duration (0-100 ms)", lower limit=0.0) -> (coerced(x)=w77:dbl)  [unwired: 1 out]
      n5 = Bundle By Name(cluster=T29 {"daqmx_channel"="", "terminal_configuration"=""} ("Pressure Control Config"), "daqmx_channel"=w92, "terminal_configuration"="RSE") -> (w109:T29)
      n6 = To Unsigned Long Integer(number=w77) -> (unsigned 32bit integer=w76:u32)
      n7 = Bundle("Pressure up", "TTL line # Pressure Up"=u8 6, w102, w102) -> (w100:T30)  [unwired: 1 in]
      n8 = Bundle("Pressure down", "TTL line # Pressure Down"=u8 8, w102, w102) -> (w101:T31)  [unwired: 1 in]
      n9 = Bundle("Pressure vacuum", "TTL line # Pressure Vacuum"=u8 7, w102, w102) -> (w99:T32)  [unwired: 1 in]
      n10 = Build Array(w100, w101, w99) -> (w98:T33)
      n11 = call "Initialize.vi"("Pulse duration (ms)"=w76, "TTL Ports"=w94, "TTL in"=refnum<class "TTL.lvclass"> refnum ("TTL.lvclass")) -> ("error out"=w97:errorcluster, "TTL out"=w86:refnum<class "TTL.lvclass">)  [unwired: 7 in]
      n12 = call "Initialize.vi"("TTL Lines"=w98, "error in (no error)"=w97, "TTL"=w86, "Pressure Control Config"=w109, "Pressure Control in"=refnum<class "Pressure Control.lvclass"> refnum ("Pressure Control.lvclass")) -> ("error out"=w114:errorcluster, "Pressure Control out"=w96:refnum<class "Pressure Control.lvclass">)  [unwired: 5 in]
      n13 = call "Get line states.vi"("error in (no error)"=w114, "TTL in"=w86) -> ("error out"=w81:errorcluster, "Current line states"=w82:bool[], "TTL out"=w85:refnum<class "TTL.lvclass">)  [unwired: 7 in]
      n14 = Array Size(array=w82) -> (size(s)=w83:i32)
      n15 = for {
        N: w83 -> [_]
        shift-right: [w120] -> w84
        shift-left: w85 -> [w121]
        shift-right: [w118] -> w115
        shift-left: w81 -> [w119]
        i -> [w117]
        n16 = call "Set line.vi"("error in (no error)"=w119, "Action"=enum16{"Open", "Close", "Toggle"}."Open", "Line number"=w117, "TTL in"=w121) -> ("error out"=w118:errorcluster, "TTL out"=w120:refnum<class "TTL.lvclass">)  [unwired: 6 in]
      }
      n17 = case shown="No Error" w115 {
        selector: w115 -> [_ w175]
        tunnel: w96 -> [w126 _]
        tunnel: w84 -> [w125 _]
        tunnel: [w122 w174] -> w89
        frame No Error {
          n18 = while {
            shift-right: [w134] -> w123
            shift-left: w126 -> [w133]
            shift-right: [w132] -> w124
            shift-left: w125 -> [w131]
            stop <- w129 stop-if-true
            n19 = call "Get pressure.vi"("Pressure Control in"=w133) -> ("Pressure"=→"Pressure":dbl)  [unwired: 7 in, 3 out]
            n20 = event shown="[7] \"Pulse Duration (0-100 ms)\": Value Change" {
              selector: _ -> [_ _ _ _ _ _ _ _]
              dyn-events: _ -> [_ _ _ _ _ _ _ _]
              timeout: 100 -> [_ _ _ _ _ _ _ _]
              tunnel: [w137 w140 w141 w146 w150 w155 w160 w172] -> w134
              tunnel: w133 -> [w137 w140 w142 w147 w151 w156 w161 w173]
              tunnel: [w136 w139 w143 w148 w152 w157 w162 w170] -> w132
              tunnel: w131 -> [w136 w139 w143 w148 w152 w157 w162 w171]
              tunnel: [_ TRUE _ _ _ _ _ _] -> w129
              tunnel: [_ _ w144 w149 w153 w158 w163 w169] -> w128
              event Timeout {
                n21 = event-data() -> ()  [unwired: 1 in, 2 out]
              }
              event "Stop All": Value Change {
                n22 = event-data() -> ()  [unwired: 1 in, 6 out]
              }
              event "Vent pressure": Value Change {
                n23 = event-data() -> ()  [unwired: 1 in, 5 out]
                n24 = call "Vent.vi"("Pressure Control in"=w142) -> ("error out"=w144:errorcluster, "Pressure Control out"=w141:refnum<class "Pressure Control.lvclass">)  [unwired: 9 in]
              }
              event "Vacuum": Value Change {
                n25 = event-data() -> ("NewVal"=w145:bool)  [unwired: 1 in, 4 out]
                n26 = call "Set vacuum.vi"("Vacuum?"=w145, "Pressure Control in"=w147) -> ("error out"=w149:errorcluster, "Pressure Control out"=w146:refnum<class "Pressure Control.lvclass">)  [unwired: 8 in]
              }
              event "Set zero pressure": Value Change {
                n27 = event-data() -> ()  [unwired: 1 in, 5 out]
                n28 = call "Set zero pressure to current pressure.vi"("Pressure Control in"=w151) -> ("error out"=w153:errorcluster, "Pressure Control out"=w150:refnum<class "Pressure Control.lvclass">)  [unwired: 8 in, 1 out]
              }
              event "Pressure Up": Value Change {
                n29 = event-data() -> ()  [unwired: 1 in, 5 out]
                n30 = call "Pressure pulse.vi"("Up or down?"=enum16{"Up", "Down"}."Up", "Pressure Control in"=w156) -> ("error out"=w158:errorcluster, "Pressure Control out"=w155:refnum<class "Pressure Control.lvclass">)  [unwired: 8 in]
              }
              event "Pressure Down": Value Change {
                n31 = event-data() -> ()  [unwired: 1 in, 5 out]
                n32 = call "Pressure pulse.vi"("Up or down?"=enum16{"Up", "Down"}."Down", "Pressure Control in"=w161) -> ("error out"=w163:errorcluster, "Pressure Control out"=w160:refnum<class "Pressure Control.lvclass">)  [unwired: 8 in]
              }
              event "Pulse Duration (0-100 ms)": Value Change {
                # "Event added by Ronen to allow for changes\nin pulse duration as program is running"
                n33 = event-data() -> ()  [unwired: 1 in, 6 out]
                n34 = local read "Pulse Duration (0-100 ms)"() -> (w167:dbl)
                n35 = In Range and Coerce(upper limit=100.0, x=w167, lower limit=0.0) -> (coerced(x)=w165:dbl)  [unwired: 1 out]
                n36 = To Unsigned Long Integer(number=w165) -> (unsigned 32bit integer=w164:u32)
                n37 = call "Change TTL - Ronen.vi"("Pulse Duration (ms)"=w164, "TTL.lvclass"=w171) -> ("error out"=w169:errorcluster, "TTL.lvclass"=w170:refnum<class "TTL.lvclass">)  [unwired: 8 in]
                n38 = call "Update TTL - Ronen.vi"("TTL.lvclass"=w170, "Pressure Control in"=w173) -> ("Pressure Control out"=w172:refnum<class "Pressure Control.lvclass">)  [unwired: 8 in, 1 out]
              }
            }
            n39 = call <vilib>:"Simple Error Handler.vi"("error in (no error)"=w128) -> ()  [unwired: 4 in, 5 out]
          }
          n40 = call "Close.vi"("Pressure Control in"=w123) -> ("error out"=w127:errorcluster)  [unwired: 9 in, 1 out]
          n41 = call "Close.vi"("error in (no error)"=w127, "TTL in"=w124) -> ("error out"=w122:errorcluster)  [unwired: 8 in, 1 out]
        }
        frame Error {
          n42 = call <vilib>:"Simple Error Handler.vi"("error in (no error)"=w175) -> ("error out"=w174:errorcluster)  [unwired: 4 in, 4 out]
        }
      }
      n43 = property on="DAQmx Device Name" class="DAQmxName"("Visible"=FALSE) -> ()  [unwired: 2 in, 2 out]
      n44 = call <vilib>:"Clear Errors.vi"("error in (no error)"=w89) -> ("error out"=w87:errorcluster)  [unwired: 5 in, 1 out]
      n45 = property on="DAQmx Device Name" class="DAQmxName"(error in=w87, "Visible"=TRUE) -> ()  [unwired: 1 in, 2 out]
    }
    frame Disabled {
    }
  }
  n46 = disable-structure shown="Disabled" {
    disable-tunnel: [w207 _] -> w55
    disable-tunnel: [w204 _] -> w44
    disable-tunnel: [w203 _] -> w43
    disable-tunnel: [w198 _] -> w39
    disable-tunnel: [w197 _] -> w38
    disable-tunnel: [w196 _] -> w37
    disable-tunnel: [w195 _] -> w36
    disable-tunnel: [w192 _] -> w28
    disable-tunnel: [w187 _] -> w9
    disable-tunnel: [w180 _] -> w8
    disable-tunnel: [w177 _] -> w7
    frame Disabled {
      w179 = u16 20 items=["1.0"=10, "1.5"=15, "2.0"=20] ("stop bits (10: 1 bit)")
      w190 = u16 20 items=["1.0"=10, "1.5"=15, "2.0"=20] ("stop bits (10: 1 bit)")
      w193 = u16 10 items=["1.0"=10, "1.5"=15, "2.0"=20] ("stop bits (10: 1 bit)")
      w199 = u16 20 items=["1.0"=10, "1.5"=15, "2.0"=20] ("stop bits (10: 1 bit)")
      w201 = u16 20 items=["1.0"=10, "1.5"=15, "2.0"=20] ("stop bits (10: 1 bit)")
      w205 = u16 20 items=["1.0"=10, "1.5"=15, "2.0"=20] ("stop bits (10: 1 bit)")
      # "Bottom 1 Harvard"
      # "Top 3 Harvard"
      # "Center Harvard"
      n47 = call-poly "VISA Configure Serial Port"("VISA resource name"=refnum<visa-resource-name> "COM2", "baud rate (9600)"=u32 9600, "stop bits (10: 1 bit)"=w190) -> ("VISA resource name out"=w180:refnum<visa-resource-name>, "error out"=→"Preamp Error Out":errorcluster)  [unwired: 4 in, 7 out]
      n48 = call-poly "VISA Configure Serial Port"("VISA resource name"=refnum<visa-resource-name> "COM2", "baud rate (9600)"=u32 9600, "stop bits (10: 1 bit)"=w179) -> ("VISA resource name out"=w177:refnum<visa-resource-name>)  [unwired: 4 in, 8 out]
      n49 = call-poly "VISA Configure Serial Port"("VISA resource name"=refnum<visa-resource-name> "COM7", "baud rate (9600)"=u32 115200, "stop bits (10: 1 bit)"=w193) -> ("VISA resource name out"=w192:refnum<visa-resource-name>, "error out"=w191:errorcluster)  [unwired: 4 in, 7 out]
      n50 = call-poly "VISA Configure Serial Port"("VISA resource name"=refnum<visa-resource-name> "COM5", "baud rate (9600)"=u32 115200, "stop bits (10: 1 bit)"=w199) -> ("VISA resource name out"=w196:refnum<visa-resource-name>, "error out"=w195:errorcluster)  [unwired: 4 in, 7 out]
      n51 = call-poly "VISA Configure Serial Port"("VISA resource name"=refnum<visa-resource-name> "COM4", "baud rate (9600)"=u32 115200, "stop bits (10: 1 bit)"=w201) -> ("VISA resource name out"=w198:refnum<visa-resource-name>, "error out"=w197:errorcluster)  [unwired: 4 in, 7 out]
      n52 = call-poly "VISA Configure Serial Port"("VISA resource name"=refnum<visa-resource-name> "COM6", "baud rate (9600)"=u32 115200, "stop bits (10: 1 bit)"=w205) -> ("VISA resource name out"=w203:refnum<visa-resource-name>, "error out"=w204:errorcluster)  [unwired: 4 in, 7 out]
      n53 = call-poly "VISA Configure Serial Port"("VISA resource name"=refnum<visa-resource-name> "COM1") -> ("VISA resource name out"=w187:refnum<visa-resource-name>, "error out"=w207:errorcluster)  [unwired: 5 in, 8 out]
      "Stage Control Serial Error" <- w207
      n54 = local write "Blue Error Out"(w191) -> ()
    }
    frame Enabled {
    }
  }
  n55 = call "IMAQ Create"("Image Name"="APD 1 Image", "Image Type"=w32) -> ("New Image"=w49:T6)  [unwired: 3 in, 1 out]
  n56 = call "IMAQ Create"("Image Name"="APD 2 Image", "Image Type"=w32) -> ("New Image"=w48:T6)  [unwired: 3 in, 1 out]
  n57 = call "IMAQ Create"("Image Name"="APD 3 Image", "Image Type"=w32) -> ("New Image"=w31:T6)  [unwired: 3 in, 1 out]
  n58 = call "IMAQ Create"("Image Name"="Det. X Image", "Image Type"=w32) -> ("New Image"=w47:T6)  [unwired: 3 in, 1 out]
  n59 = call "IMAQ Create"("Image Name"="Det. Y Image", "Image Type"=w32) -> ("New Image"=w46:T6)  [unwired: 3 in, 1 out]
